vi "VISA Read Async.vi"(8 "error in (no error)":errorcluster, 10 "byte count":u32, 11 "Instrument in":refnum<class "Instrument.lvclass">) -> (0 "error out":errorcluster, 1 "return count":u32, 2 "read buffer":string, 3 "Instrument out":refnum<class "Instrument.lvclass">)   [LabVIEW 2017, in "Instrument.lvclass"]
doc: "(Dynamic) Read from this Instrument using an asynchronous VISA call. Override this method if the Instrument has communication idiosyncrasies."
uses:
  Instrument.lvclass
  Instrument.lvclass/Instrument.ctl
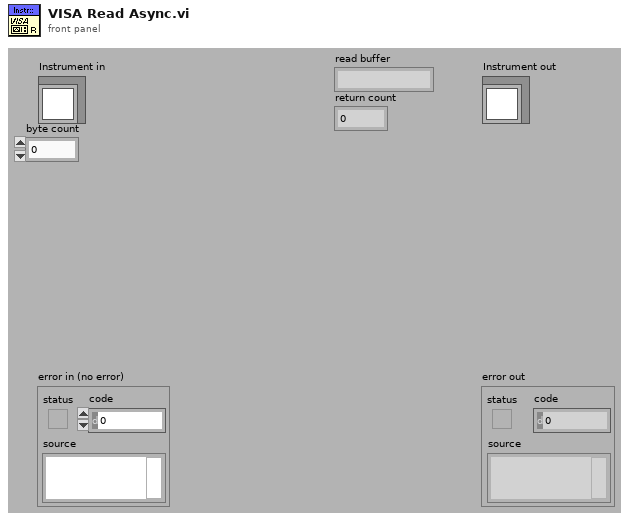
[diagram p1: front panel]
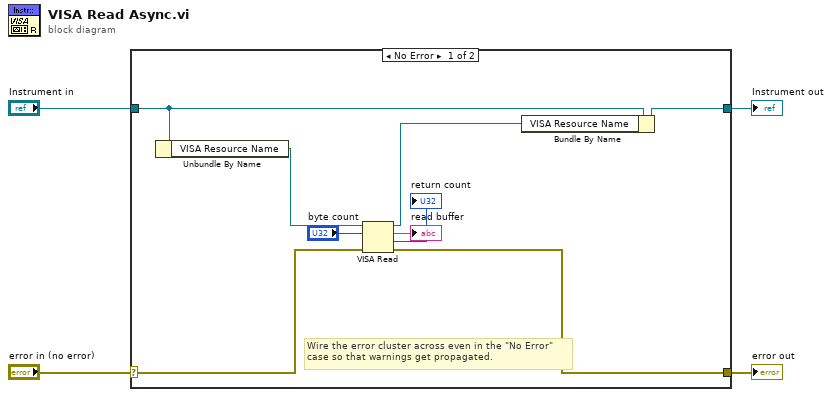
[diagram p0: block diagram]
diagram:
  n1 = case shown="No Error" "error in (no error)" {
    selector: "error in (no error)" -> [w13 w15]
    tunnel: [w12 w15] -> w3
    tunnel: [w9 w14] -> w1
    tunnel: "Instrument in" -> [w11 w14]
    frame No Error {
      # "Wire the error cluster across even in the \"No Error\"\ncase so that warnings get propagated."
      n2 = Unbundle By Name(w11) -> ("VISA Resource Name"=w10:refnum<visa-resource-name>)
      n3 = VISA Read(VISA resource name=w10, byte count="byte count", error in (no error)=w13) -> (VISA resource name out=w8:refnum<visa-resource-name>, read buffer=→"read buffer":string, return count=→"return count":u32, error out=w12:errorcluster)
      n4 = Bundle By Name(cluster=w11, "VISA Resource Name"=w8) -> (w9:refnum<class "Instrument.lvclass">)
    }
    frame Error {
    }
  }
  "error out" <- w3
  "Instrument out" <- w1
